vi "Read Controls from Config File.vi"(6 "Child?":bool, 7 "section":string, 8 "Error In":errorcluster, 9 "ParentName":string, 10 "Ctl Refnum":refnum<vi>, 11 "refnum":T1) -> (0 "Error Out":errorcluster, 3 "refnum out":T1)   [LabVIEW 2018]
uses:
  <vilib>/Utility/config.llb/Config Data RefNum.ctl
  Hardware Mfg/Thorlabs Translation Stages/Controls/Translation Stage Cluster.ctl
  Controls/Translation Stage Types.ctl
  <vilib>/Utility/config.llb/Read Key (String).vi
  <vilib>/Utility/config.llb/Read Key (Boolean).vi
  <vilib>/Utility/config.llb/Read Key (Double).vi
  <vilib>/Utility/config.llb/Read Key (U32).vi
  <vilib>/Utility/config.llb/NI_LVConfig.lvlib
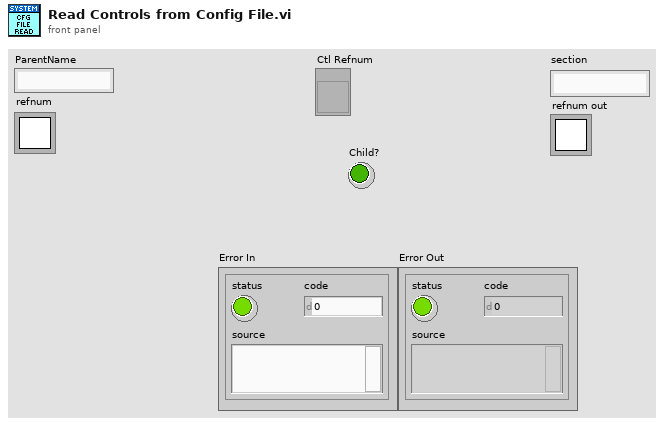
[diagram p1: front panel]
types:
  T1 = typedef "NI_LVConfig.lvlib/Config Data RefNum.ctl" = refnum<k1>
  T2 = typedef "Translation Stage Cluster.ctl" = cluster{"Position":dbl, "Is.Enabled?":bool, "Is.Connected?":bool, "Device SN":string, "AccelerationMaximum":dbl, "VelocityMaximum":dbl, "Acceleration":dbl, "Velocity":dbl, "waitTimeout (ms)":i32, "Model":T3, "Is.Homed?":bool, "MOVE":bool}
  T3 = typedef "Translation Stage Types.ctl" = enum16{"None", "Thorlabs LTS", "Thorlabs MLJ"}
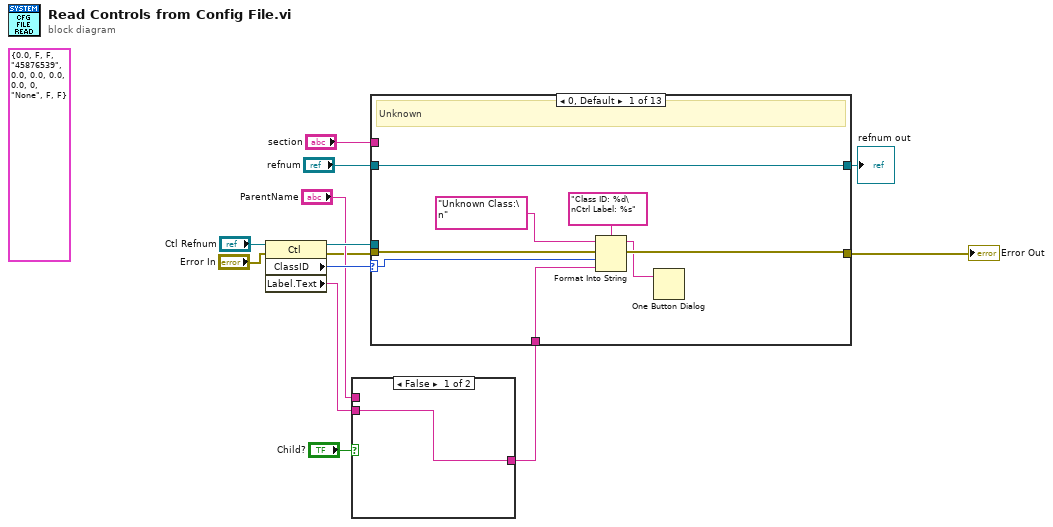
[diagram p0: block diagram]
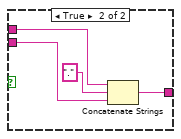
[diagram p2: hidden frame]
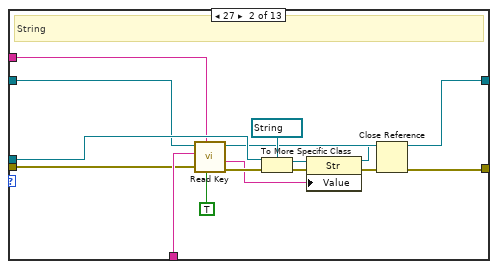
[diagram p3: hidden frame]
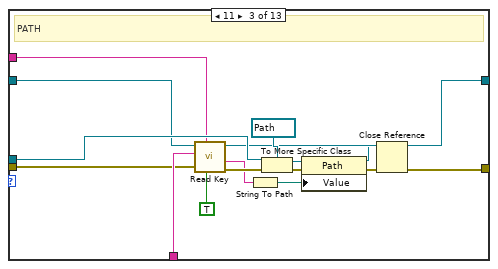
[diagram p4: hidden frame]
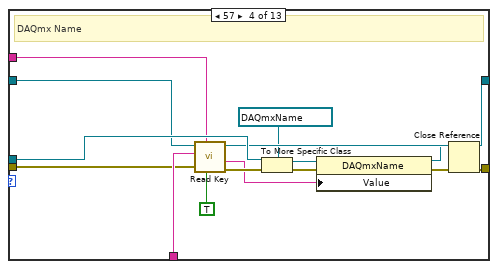
[diagram p5: hidden frame]
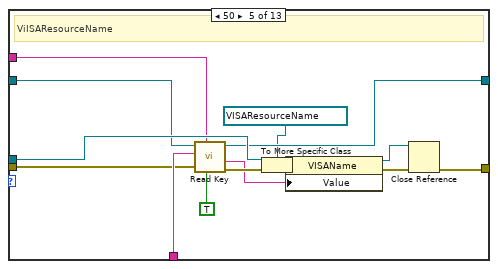
[diagram p6: hidden frame]
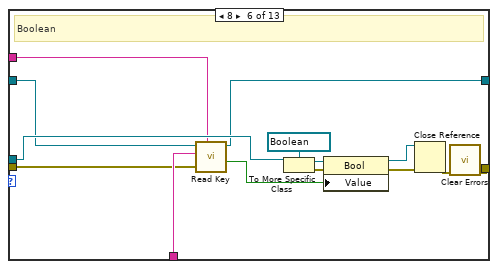
[diagram p7: hidden frame]
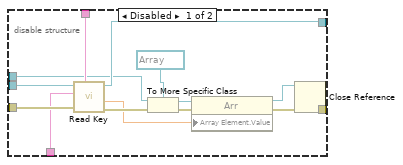
[diagram p9: hidden frame]
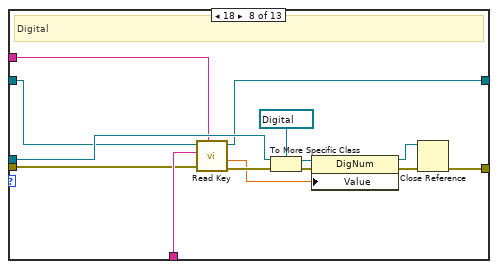
[diagram p10: hidden frame]
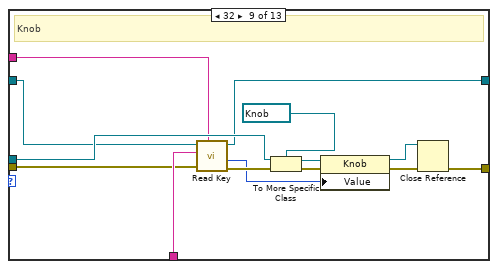
[diagram p11: hidden frame]
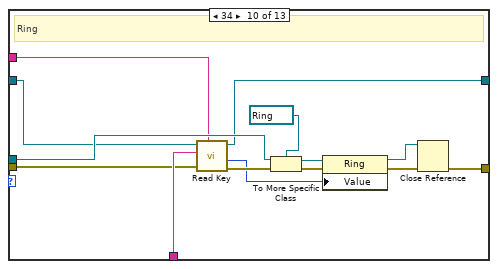
[diagram p12: hidden frame]
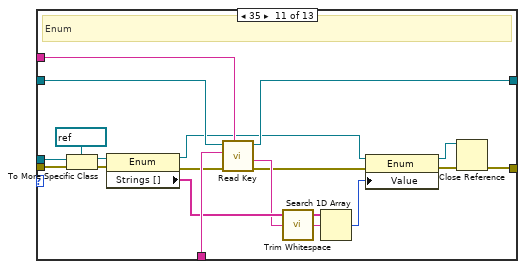
[diagram p13: hidden frame]
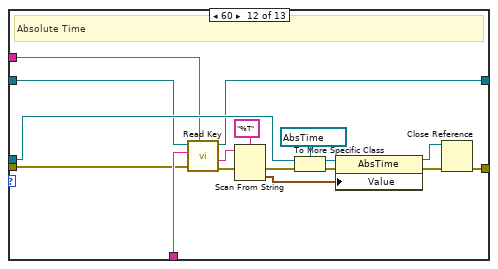
[diagram p14: hidden frame]
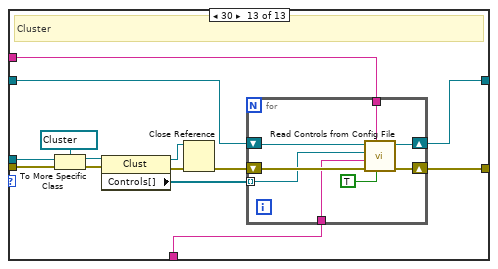
[diagram p15: hidden frame]
diagram:
  (unwired) T2 {"Position"=0.0, "Is.Enabled?"=FALSE, "Is.Connected?"=FALSE, "Device SN"="45876539", "AccelerationMaximum"=0.0, "VelocityMaximum"=0.0, "Acceleration"=0.0, "Velocity"=0.0, "waitTimeout (ms)"=0, "Model"=enum."None", "Is.Homed?"=FALSE, "MOVE"=FALSE} ("Control Param In")
  n1 = property class="Ctl"(reference="Ctl Refnum", error in="Error In") -> (reference out=w12:refnum<vi>, error out=w6:errorcluster, "ClassID"=w11:u32, "Label.Text"=w8:string)
  n2 = case shown="False" "Child?" {
    tunnel: "ParentName" -> [_ w18]
    tunnel: w8 -> [w14 w16]
    tunnel: [w14 w15] -> w3
    frame False {
    }
    frame True {
      n3 = Concatenate Strings(w18, ".", w16) -> (w15:string)
    }
  }
  n4 = case shown="0, Default" w11 {
    selector: w11 -> [w23 _ _ _ _ _ _ _ _ _ _ _ _]
    tunnel: w6 -> [w21 w30 w46 w62 w77 w91 w107 w127 w142 w156 w185 w191 w216]
    tunnel: w12 -> [_ w40 w56 w72 w87 w100 w102 w138 w152 w166 w184 w202 w214]
    tunnel: [w20 w28 w44 w60 w75 w88 w106 w128 w143 w157 w168 w192 w210] -> w1
    tunnel: "section" -> [_ w39 w55 w71 w86 w99 w108 w131 w146 w160 w180 w196 w207]
    tunnel: "refnum" -> [w26 w38 w54 w70 w85 w98 w103 w130 w145 w159 w179 w195 w209]
    tunnel: [w26 w37 w53 w69 w84 w97 w105 w129 w144 w158 w178 w194 w208] -> w2
    tunnel: w3 -> [w22 w35 w51 w67 w82 w95 w104 w132 w147 w161 w181 w197 w206]
    frame 0, Default {
      # "Unknown"
      n5 = Format Into String(format string="Class ID: %d\nCtrl Label: %s", initial string="Unknown Class:\n" ("string"), error in=w21, w23, w22) -> (resulting string=w19:string, error out=w20:errorcluster)
      n6 = One Button Dialog(message=w19) -> ()  [unwired: 1 in, 1 out]
    }
    frame 27 {
      # "String"
      n7 = call-poly <vilib>:"Read Key.vi"("read raw string? (F)"=TRUE, "section"=w39, "error in (no error)"=w30, "key"=w35, "refnum"=w38) -> ("error out"=w29:errorcluster, "value"=w27:string, "refnum out"=w37:T1)  [unwired: 3 in, 1 out]
      n8 = To More Specific Class(target class=refnum<vi> refnum ("AccelerationMaximum 2"), reference=w40, error in=w29) -> (specific class reference=w33:refnum<vi>, error out=w36:errorcluster)
      n9 = property class="Str"(reference=w33, error in=w36, "Value"=w27) -> (reference out=w32:refnum<vi>, error out=w34:errorcluster)
      n10 = Close Reference(reference=w32, error in (no error)=w34) -> (error out=w28:errorcluster)
    }
    frame 11 {
      # "PATH"
      n11 = call-poly <vilib>:"Read Key.vi"("read raw string? (F)"=TRUE, "section"=w55, "error in (no error)"=w46, "key"=w51, "refnum"=w54) -> ("error out"=w45:errorcluster, "value"=w43:string, "refnum out"=w53:T1)  [unwired: 3 in, 1 out]
      n12 = String To Path(string=w43) -> (path=w42:path)
      n13 = To More Specific Class(target class=refnum<vi> refnum ("AccelerationMaximum 2"), reference=w56, error in=w45) -> (specific class reference=w49:refnum<vi>, error out=w52:errorcluster)
      n14 = property class="Path"(reference=w49, error in=w52, "Value"=w42) -> (reference out=w48:refnum<vi>, error out=w50:errorcluster)
      n15 = Close Reference(reference=w48, error in (no error)=w50) -> (error out=w44:errorcluster)
    }
    frame 57 {
      # "DAQmx Name"
      n16 = call-poly <vilib>:"Read Key.vi"("read raw string? (F)"=TRUE, "section"=w71, "error in (no error)"=w62, "key"=w67, "refnum"=w70) -> ("error out"=w61:errorcluster, "value"=w59:string, "refnum out"=w69:T1)  [unwired: 3 in, 1 out]
      n17 = To More Specific Class(target class=refnum<vi> refnum ("Analog Out Channel"), reference=w72, error in=w61) -> (specific class reference=w65:refnum<vi>, error out=w68:errorcluster)
      n18 = property class="DAQmxName"(reference=w65, error in=w68, "Value"=w59) -> (reference out=w64:refnum<vi>, error out=w66:errorcluster)
      n19 = Close Reference(reference=w64, error in (no error)=w66) -> (error out=w60:errorcluster)
    }
    frame 50 {
      # "ViISAResourceName"
      n20 = call-poly <vilib>:"Read Key.vi"("read raw string? (F)"=TRUE, "section"=w86, "error in (no error)"=w77, "key"=w82, "refnum"=w85) -> ("error out"=w76:errorcluster, "value"=w74:string, "refnum out"=w84:T1)  [unwired: 3 in, 1 out]
      n21 = To More Specific Class(target class=refnum<vi> refnum ("Controller VISA Ref"), reference=w87, error in=w76) -> (specific class reference=w80:refnum<vi>, error out=w83:errorcluster)
      n22 = property class="VISAName"(reference=w80, error in=w83, "Value"=w74) -> (reference out=w79:refnum<vi>, error out=w81:errorcluster)
      n23 = Close Reference(reference=w79, error in (no error)=w81) -> (error out=w75:errorcluster)
    }
    frame 8 {
      # "Boolean"
      n24 = call-poly <vilib>:"Read Key.vi"("section"=w99, "error in (no error)"=w91, "key"=w95, "refnum"=w98) -> ("value"=w90:bool, "refnum out"=w97:T1)  [unwired: 4 in, 2 out]
      n25 = To More Specific Class(target class=refnum<vi> refnum ("AccelerationMaximum 2"), reference=w100) -> (specific class reference=w93:refnum<vi>, error out=w96:errorcluster)  [unwired: 1 in]
      n26 = property class="Bool"(reference=w93, error in=w96, "Value"=w90) -> (reference out=w92:refnum<vi>, error out=w94:errorcluster)
      n27 = Close Reference(reference=w92, error in (no error)=w94) -> (error out=w89:errorcluster)
      n28 = call <vilib>:"Clear Errors.vi"("error in (no error)"=w89) -> ("error out"=w88:errorcluster)  [unwired: 5 in, 1 out]
    }
    frame 14 {
      n29 = disable-structure shown="Enabled" {
        disable-tunnel: w108 -> [w115 _]
        disable-tunnel: w107 -> [w114 w124]
        disable-tunnel: [w113 w124] -> w106
        disable-tunnel: [w112 w123] -> w105
        disable-tunnel: w104 -> [w111 _]
        disable-tunnel: w103 -> [w110 w123]
        disable-tunnel: w102 -> [w109 _]
        frame Disabled {
          n30 = call-poly <vilib>:"Read Key.vi"("section"=w115, "error in (no error)"=w114, "key"=w111, "refnum"=w110) -> ("error out"=w117:errorcluster, "value"=w116:dbl, "refnum out"=w112:T1)  [unwired: 4 in, 1 out]
          n31 = To More Specific Class(target class=refnum<vi> refnum ("AccelerationMaximum 2"), reference=w109, error in=w117) -> (specific class reference=w120:refnum<vi>, error out=w121:errorcluster)
          n32 = property class="Arr"(reference=w120, error in=w121, "Array Element.Value"=w116) -> (reference out=w118:refnum<vi>, error out=w119:errorcluster)
          n33 = Close Reference(reference=w118, error in (no error)=w119) -> (error out=w113:errorcluster)
        }
        frame Enabled {
        }
      }
    }
    frame 18 {
      # "Digital"
      n34 = call-poly <vilib>:"Read Key.vi"("section"=w131, "error in (no error)"=w127, "key"=w132, "refnum"=w130) -> ("error out"=w126:errorcluster, "value"=w125:dbl, "refnum out"=w129:T1)  [unwired: 4 in, 1 out]
      n35 = To More Specific Class(target class=refnum<vi> refnum ("AccelerationMaximum 2"), reference=w138, error in=w126) -> (specific class reference=w135:refnum<vi>, error out=w136:errorcluster)
      n36 = property class="DigNum"(reference=w135, error in=w136, "Value"=w125) -> (reference out=w133:refnum<vi>, error out=w134:errorcluster)
      n37 = Close Reference(reference=w133, error in (no error)=w134) -> (error out=w128:errorcluster)
    }
    frame 32 {
      # "Knob"
      n38 = call-poly <vilib>:"Read Key.vi"("section"=w146, "error in (no error)"=w142, "key"=w147, "refnum"=w145) -> ("error out"=w141:errorcluster, "value"=w140:u32, "refnum out"=w144:T1)  [unwired: 4 in, 1 out]
      n39 = To More Specific Class(target class=refnum<vi> refnum ("Zoom Factor"), reference=w152, error in=w141) -> (specific class reference=w150:refnum<vi>, error out=w151:errorcluster)
      n40 = property class="Knob"(reference=w150, error in=w151, "Value"=w140) -> (reference out=w148:refnum<vi>, error out=w149:errorcluster)
      n41 = Close Reference(reference=w148, error in (no error)=w149) -> (error out=w143:errorcluster)
    }
    frame 34 {
      # "Ring"
      n42 = call-poly <vilib>:"Read Key.vi"("section"=w160, "error in (no error)"=w156, "key"=w161, "refnum"=w159) -> ("error out"=w155:errorcluster, "value"=w154:u32, "refnum out"=w158:T1)  [unwired: 4 in, 1 out]
      n43 = To More Specific Class(target class=refnum<vi> refnum ("Trigger Operation"), reference=w166, error in=w155) -> (specific class reference=w164:refnum<vi>, error out=w165:errorcluster)
      n44 = property class="Ring"(reference=w164, error in=w165, "Value"=w154) -> (reference out=w162:refnum<vi>, error out=w163:errorcluster)
      n45 = Close Reference(reference=w162, error in (no error)=w163) -> (error out=w157:errorcluster)
    }
    frame 35 {
      # "Enum"
      n46 = To More Specific Class(target class=refnum<vi> refnum ("Enum"), reference=w184, error in=w185) -> (specific class reference=w182:refnum<vi>, error out=w183:errorcluster)
      n47 = property class="Enum"(reference=w182, error in=w183) -> (reference out=w169:refnum<vi>, error out=w175:errorcluster, "Strings []"=w176:string[])
      n48 = call-poly <vilib>:"Read Key.vi"("section"=w180, "error in (no error)"=w175, "key"=w181, "refnum"=w179) -> ("error out"=w173:errorcluster, "value"=w174:string, "refnum out"=w178:T1)  [unwired: 4 in, 1 out]
      n49 = call <vilib>:"Trim Whitespace.vi"("string"=w174) -> ("trimmed string"=w171:string)  [unwired: 1 in]
      n50 = Search 1D Array(1D array=w176, element=w171) -> (index of element=w170:i32)  [unwired: 1 in]
      n51 = property class="Enum"(reference=w169, error in=w173, "Value"=w170) -> (reference out=w167:refnum<vi>, error out=w172:errorcluster)
      n52 = Close Reference(reference=w167, error in (no error)=w172) -> (error out=w168:errorcluster)
    }
    frame 60 {
      # "Absolute Time"
      n53 = call-poly <vilib>:"Read Key.vi"("section"=w196, "error in (no error)"=w191, "key"=w197, "refnum"=w195) -> ("error out"=w189:errorcluster, "value"=w186:string, "refnum out"=w194:T1)  [unwired: 4 in, 1 out]
      n54 = Scan From String(format string="%T", input string=w186, error in=w189) -> (error out=w188:errorcluster, output 1=w187:timestamp)  [unwired: 2 in, 2 out]
      n55 = To More Specific Class(target class=refnum<vi> refnum ("AccelerationMaximum 2"), reference=w202, error in=w188) -> (specific class reference=w200:refnum<vi>, error out=w201:errorcluster)
      n56 = property class="AbsTime"(reference=w200, error in=w201, "Value"=w187) -> (reference out=w198:refnum<vi>, error out=w199:errorcluster)
      n57 = Close Reference(reference=w198, error in (no error)=w199) -> (error out=w192:errorcluster)
    }
    frame 30 {
      # "Cluster"
      n58 = To More Specific Class(target class=refnum<vi> refnum ("Cluster Ref In"), reference=w214, error in=w216) -> (specific class reference=w212:refnum<vi>, error out=w213:errorcluster)
      n59 = property class="Clust"(reference=w212, error in=w213) -> (reference out=w204:refnum<vi>, error out=w211:errorcluster, "Controls[]"=w203:refnum<vi>[])
      n60 = Close Reference(reference=w204, error in (no error)=w211) -> (error out=w205:errorcluster)
      n61 = for {
        tunnel: w207 -> [w220]
        tunnel: w206 -> [w219]
        shift-right: [w223] -> w210
        shift-left: w205 -> [w224]
        shift-right: [w221] -> w208
        shift-left: w209 -> [w222]
        tunnel: w203 -> [w217] mode=indexing
        n62 = call "Read Controls from Config File.vi"("Child?"=TRUE, "section"=w220, "Error In"=w224, "ParentName"=w219, "Ctl Refnum"=w217, "refnum"=w222) -> ("Error Out"=w223:errorcluster, "refnum out"=w221:T1)  [unwired: 4 in]
      }
    }
  }
  "Error Out" <- w1
  "refnum out" <- w2
